vi "State Complete.vi"(11 "error in (no error)":errorcluster) -> (3 "Done?":bool=TRUE)   [LabVIEW 2023]
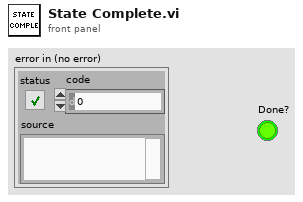
[diagram p1: front panel]
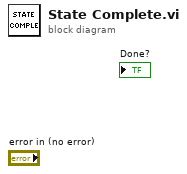
[diagram p0: block diagram]
diagram:
